vi "pneumatic control.vi"() -> ()   [LabVIEW 2018]
uses:
  <vilib>/Utility/error.llb/DialogType.ctl
  <vilib>/DAQmx/write.llb/DAQmx Write (Analog DBL 1Chan 1Samp).vi
  <vilib>/DAQmx/write.llb/DAQmx Write (Analog 1D DBL NChan 1Samp).vi
  <vilib>/DAQmx/create/channels.llb/DAQmx Create Channel (AO-Voltage-Basic).vi
  <vilib>/DAQmx/miscellaneous.llb/DAQmx Fill In Error Info.vi
panel:
  in  "水平指针滑动杆1-4":dbl(slide) scale=0.0..10.0
  in  "最大值 5":dbl=10.0 format="%0.2f"
  in  "无极控制停止按钮 1-4":bool
  in  "释放 1-4":bool
  in  "抓取1-4":bool
  in  "maximum value 6":dbl=10.0 caption="最大值" format="%0.2f"
  in  "抓放控制停止按钮1-4":bool
  in  "启用抓取控制1-4":bool
  in  "启用无极控制 1-4":bool
  in  "选项卡控件":enum32{"1-2-3", "1-3-4"}(tab)
  in  "水平指针滑动杆1-2-3":dbl(slide) scale=0.0..10.0
  in  "最大值 7":dbl=10.0 format="%0.2f"
  in  "无极控制停止按钮 1-2-3":bool
  in  "释放 1-2-3":bool
  in  "抓取1-2-3":bool
  in  "maximum value 8":dbl=10.0 caption="最大值" format="%0.2f"
  in  "抓放控制停止按钮1-2-3":bool
  in  "启用抓取控制1-2-3":bool
  in  "启用无极控制 1-2-3":bool
  in  "启用无极控制 1-3-4":bool
  in  "启用抓取控制1-3-4":bool
  in  "抓放控制停止按钮1-3-4":bool
  in  "maximum value 7":dbl=10.0 caption="最大值" format="%0.2f"
  in  "抓取1-3-4":bool
  in  "释放 1-3-4":bool
  in  "无极控制停止按钮 1-3-4":bool
  in  "最大值 6":dbl=10.0 format="%0.2f"
  in  "水平指针滑动杆1-3-4":dbl(slide) scale=0.0..10.0
  in  "水平指针滑动杆 4":dbl(slide) scale=0.0..10.0
  in  "最大值 4":dbl=10.0 format="%0.2f"
  in  "无极控制停止按钮 4":bool
  in  "释放 4":bool
  in  "抓取 4":bool
  in  "maximum value 5":dbl=10.0 caption="最大值" format="%0.2f"
  in  "抓放控制停止按钮 4":bool
  in  "启用抓取控制 4":bool
  in  "启用无极控制 4":bool
  in  "水平指针滑动杆 3":dbl(slide) scale=0.0..10.0
  in  "最大值 3":dbl=10.0 format="%0.2f"
  in  "无极控制停止按钮 3":bool
  in  "释放 3":bool
  in  "抓取 3":bool
  in  "maximum value 4":dbl=10.0 caption="最大值" format="%0.2f"
  in  "抓放控制停止按钮 3":bool
  in  "启用抓取控制 3":bool
  in  "启用无极控制 3":bool
  in  "水平指针滑动杆 2":dbl(slide) scale=0.0..10.0
  in  "最大值 2":dbl=10.0 format="%0.2f"
  in  "无极控制停止按钮 2":bool
  in  "释放 2":bool
  in  "抓取 2":bool
  in  "maximum value 3":dbl=10.0 caption="最大值" format="%0.2f"
  in  "抓放控制停止按钮 2":bool
  in  "启用抓取控制 2":bool
  in  "启用无极控制 2":bool
  in  "水平指针滑动杆":dbl(slide) scale=0.0..10.0
  in  "最大值":dbl=10.0 format="%0.2f"
  in  "无极控制停止按钮":bool
  in  "释放":bool
  in  "抓取":bool
  in  "maximum value 2":dbl=10.0 caption="最大值" format="%0.2f"
  in  "抓放控制停止按钮":bool
  in  "启用抓取控制":bool
  in  "启用无极控制":bool
  in  "总停止按钮":bool
  # "机械手驱动控制"
  # "机械手1抓放控制"
  # "机械手1滑条无极控制"
  # "机械手2抓放控制"
  # "机械手2滑条无极控制"
  # "机械手3抓放控制"
  # "机械手3滑条无极控制"
  # "机械手4抓放控制"
  # "机械手4滑条无极控制"
  # "机械手组合控制"
  # "机械手(1-4)一键控制"
  # "机械手抓放控制"
  # "机械手滑条无极控制"
  # "注意：\n  1、该模块共有“抓放控制”、“滑条无极控制”两种种机械手控制器。\n  2、点击任意控制器框内“启用X”按键即可启动该控制器，若需要切换控制器则需要先按下前面使用控制器“停止X”按键再按“启用X”按键。"
  # "机械手抓放控制"
  # "机械手滑条无极控制"
  # "机械手抓放控制"
  # "机械手滑条无极控制"
  # "4"
  # "3"
  # "2"
  # "1"
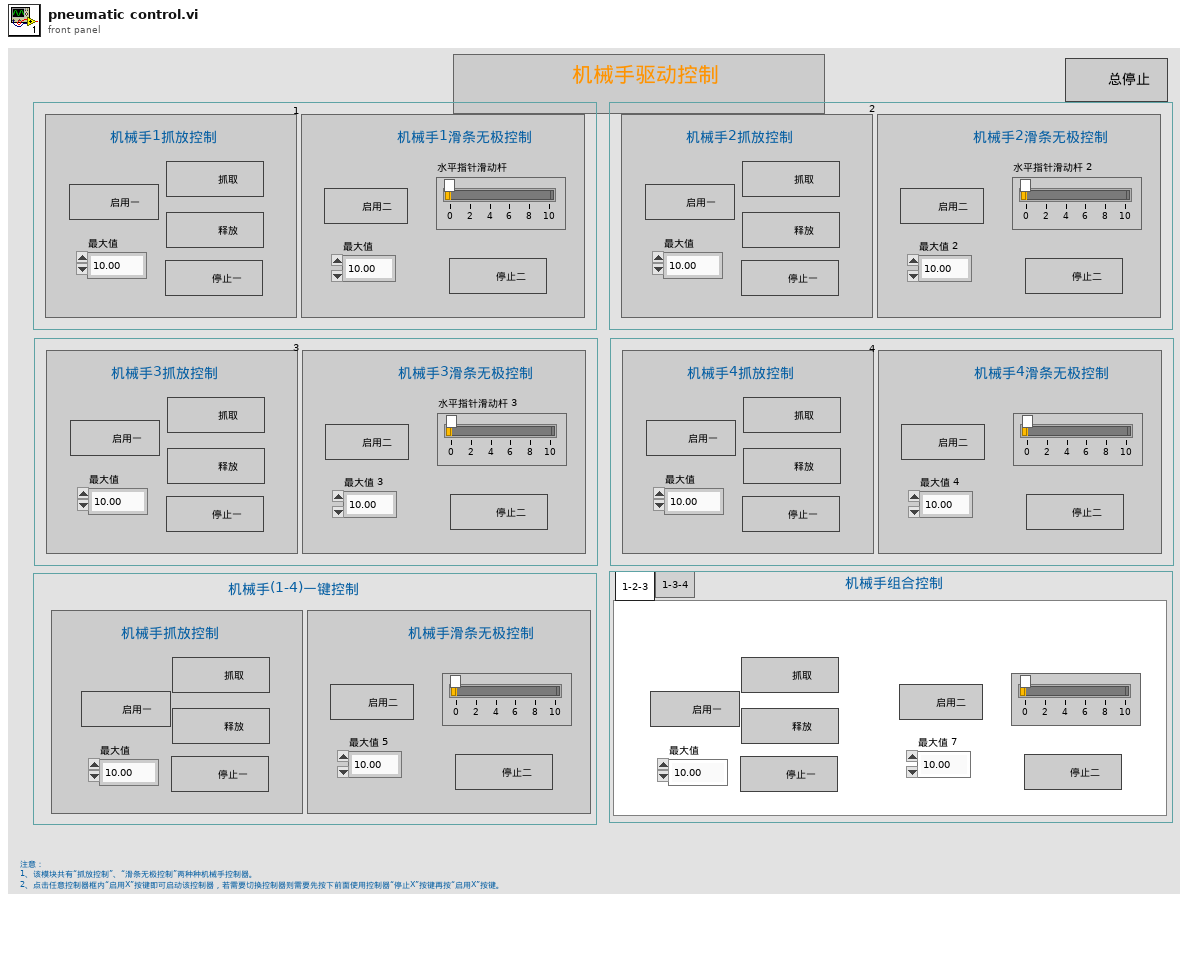
[diagram p1: front panel]
types:
  T1 = typedef "DialogType.ctl" = u16
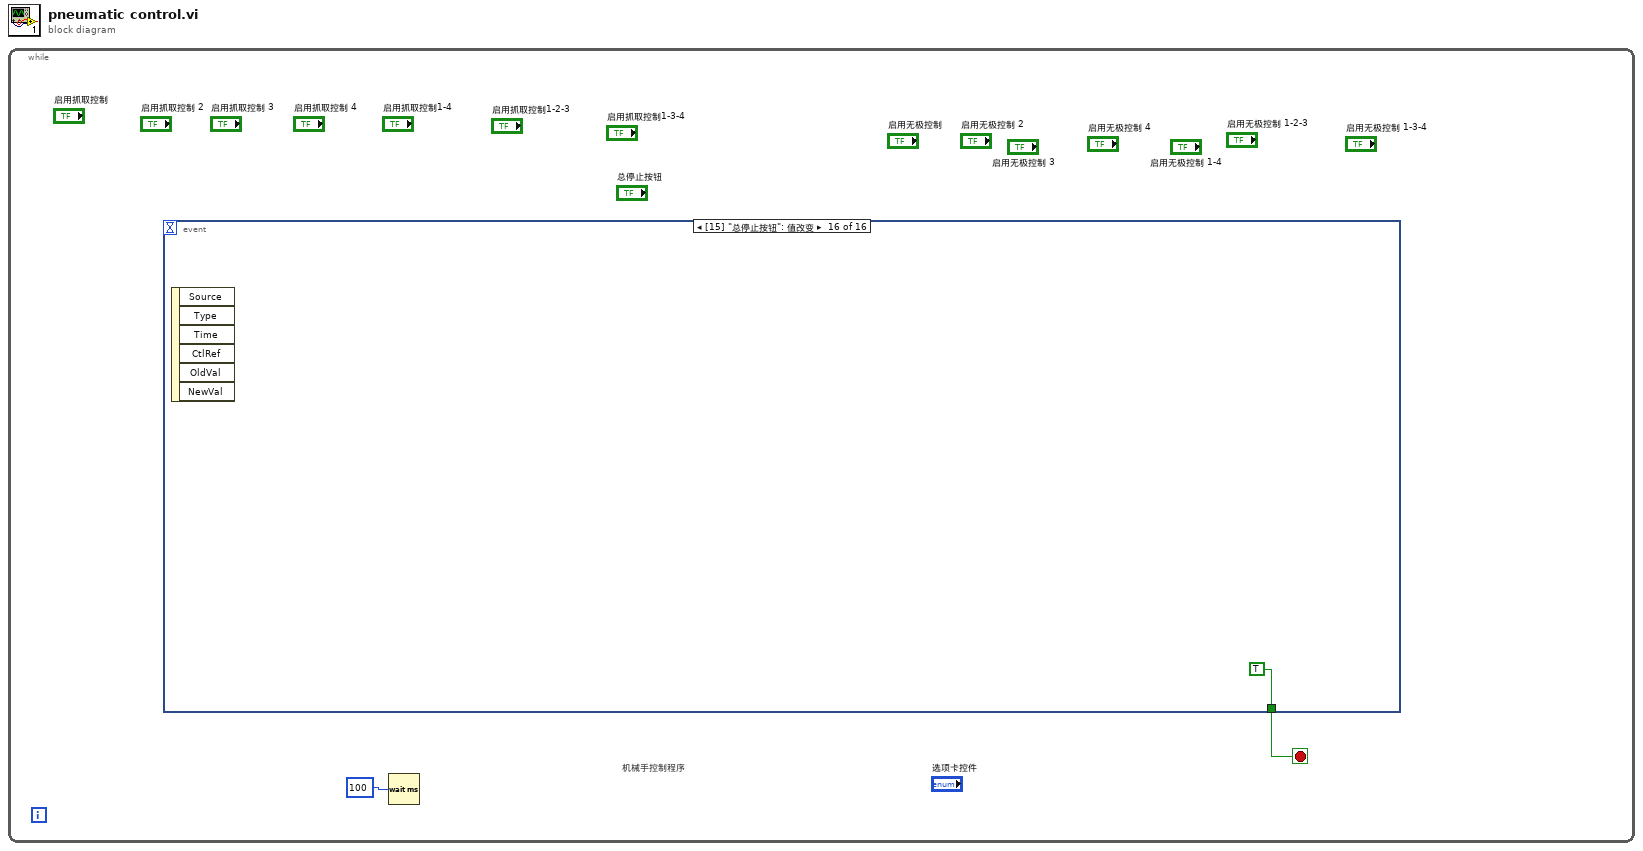
[diagram p0: block diagram]
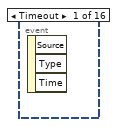
[diagram p2: hidden frame]
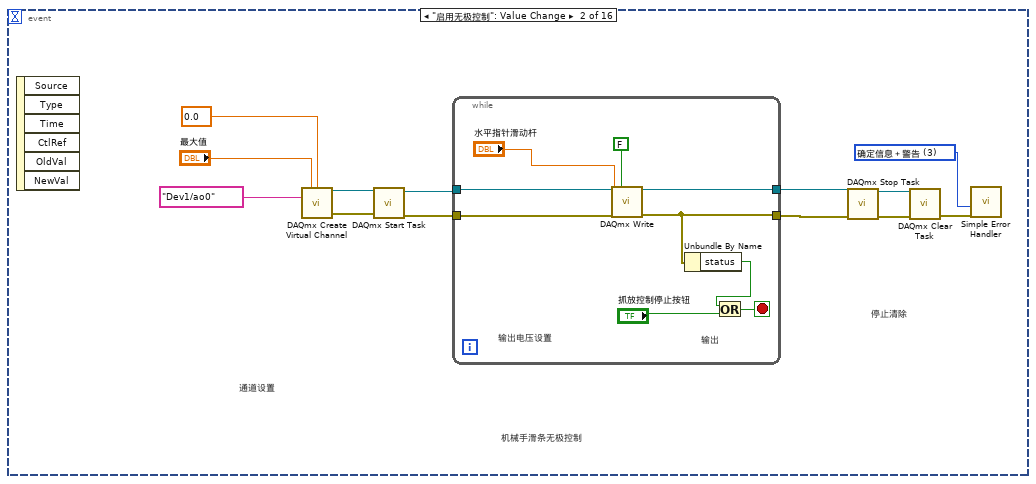
[diagram p3: hidden frame]
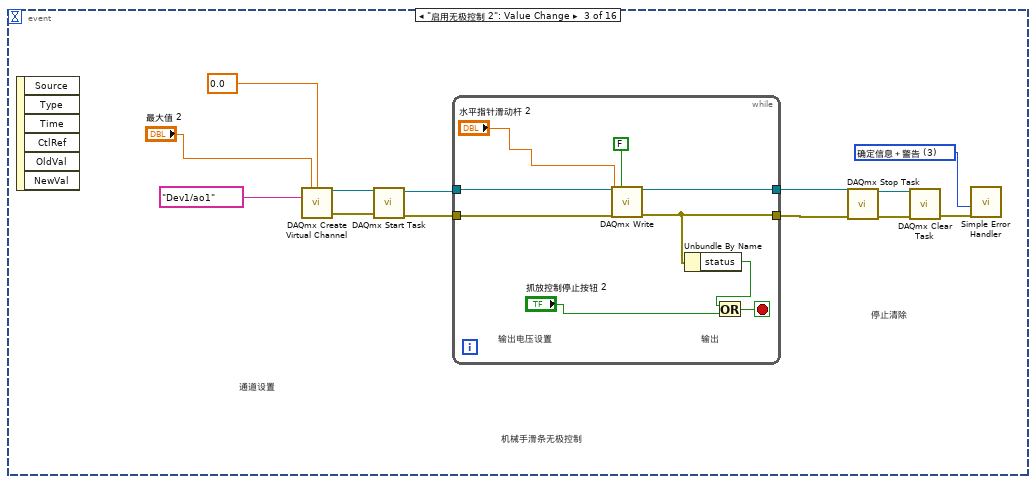
[diagram p4: hidden frame]
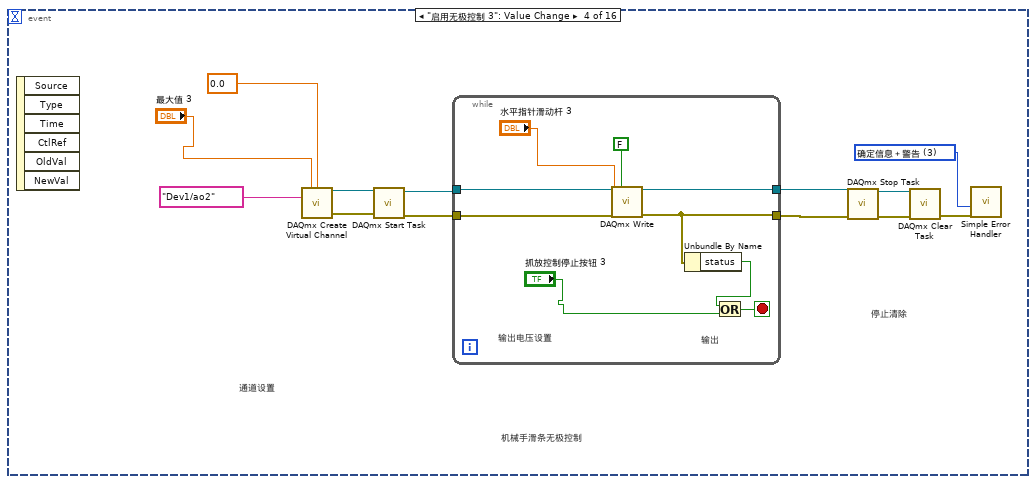
[diagram p5: hidden frame]
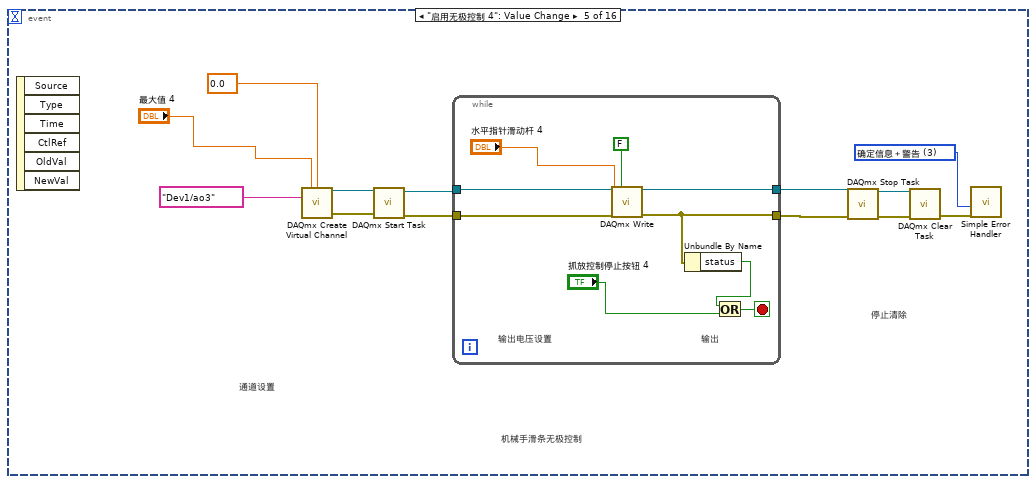
[diagram p6: hidden frame]
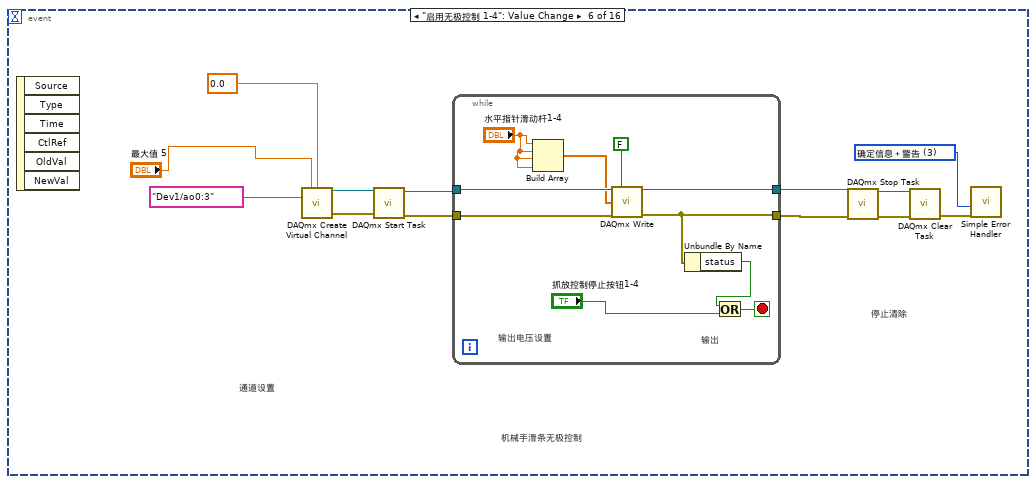
[diagram p7: hidden frame]
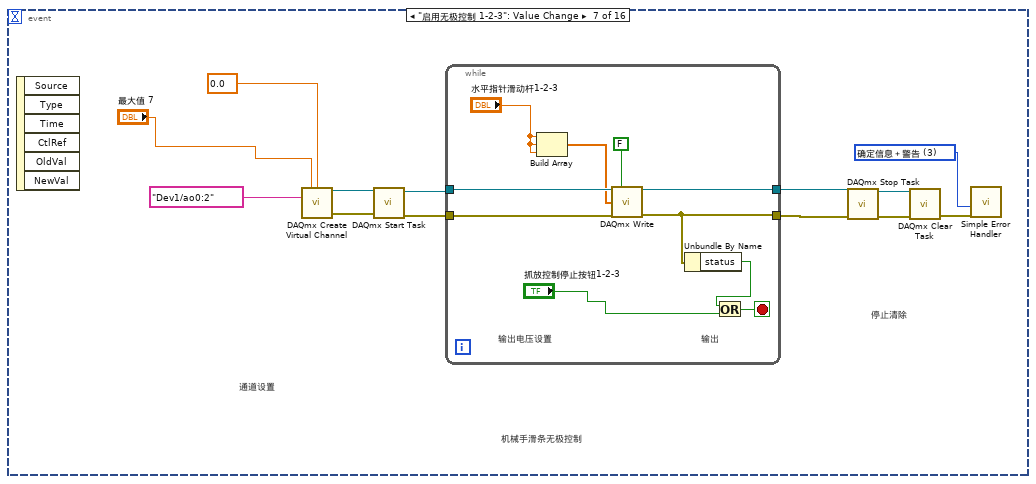
[diagram p8: hidden frame]
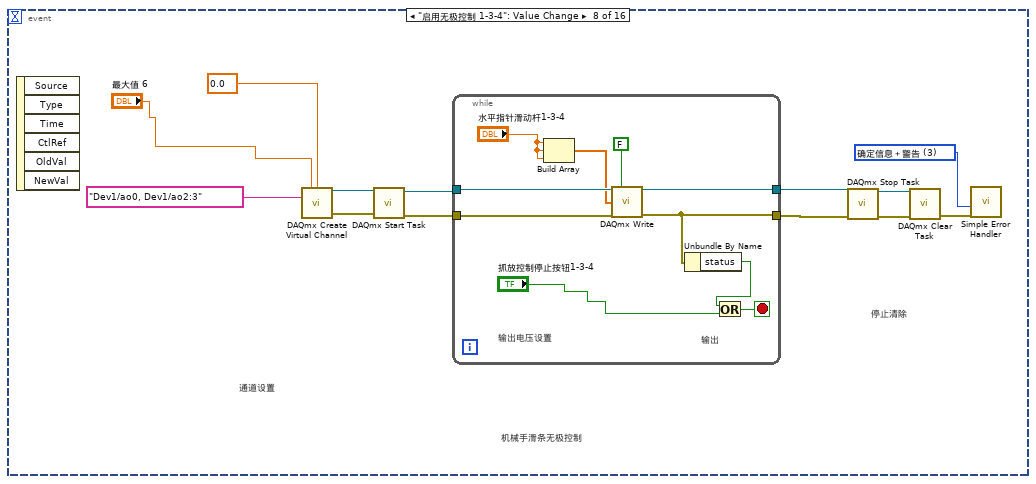
[diagram p9: hidden frame]
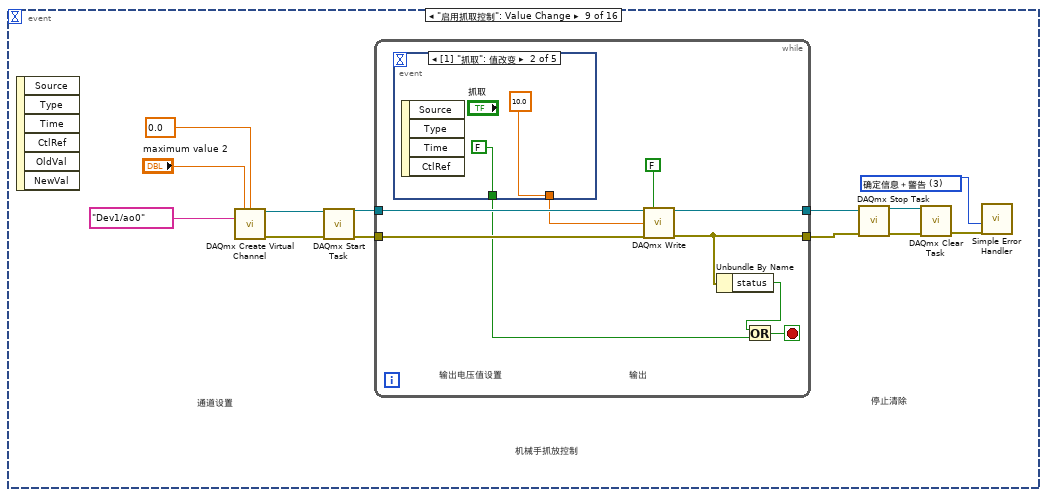
[diagram p10: hidden frame]
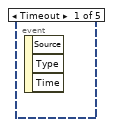
[diagram p11: hidden frame]
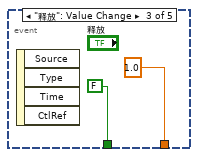
[diagram p12: hidden frame]
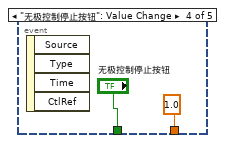
[diagram p13: hidden frame]
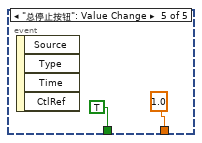
[diagram p14: hidden frame]
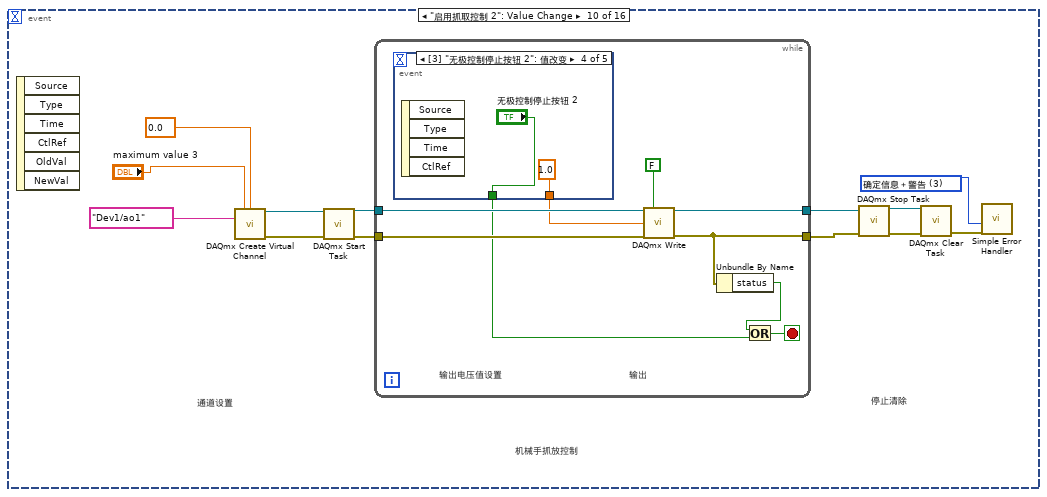
[diagram p15: hidden frame]
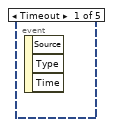
[diagram p16: hidden frame]
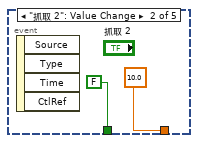
[diagram p17: hidden frame]
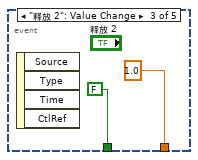
[diagram p18: hidden frame]
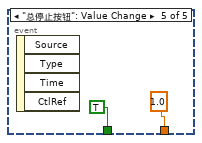
[diagram p19: hidden frame]
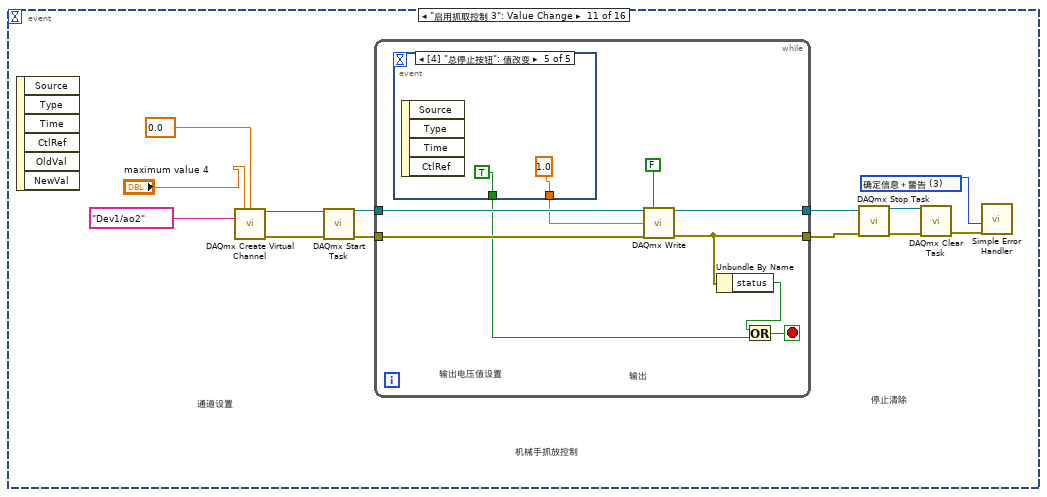
[diagram p20: hidden frame]
diagram:
  n1 = while {
    stop <- w1 stop-if-true
    # "机械手控制程序"
    n2 = event shown="[15] \"总停止按钮\": 值改变" {
      selector: _ -> [_ _ _ _ _ _ _ _ _ _ _ _ _ _ _ _]
      dyn-events: _ -> [_ _ _ _ _ _ _ _ _ _ _ _ _ _ _ _]
      timeout: _ -> [_ _ _ _ _ _ _ _ _ _ _ _ _ _ _ _]
      tunnel: [_ _ _ _ _ _ _ _ _ _ _ _ _ _ _ TRUE] -> w1
      event Timeout {
        n3 = event-data() -> ()  [unwired: 1 in, 3 out]
      }
      event "启用无极控制": Value Change {
        w4 = T1 3 items=["无对话框", "确定信息", "继续或停止信息", "确定信息＋警告", "继续/停止＋警告"] ("对话框类型（确定信息：1）")
        # "停止清除"
        # "通道设置"
        # "机械手滑条无极控制"
        n4 = event-data() -> ()  [unwired: 1 in, 6 out]
        n5 = call-poly <vilib>:"DAQmx Create Virtual Channel.vi"("maximum value"="最大值", "minimum value"=0.0, "physical channels"=tag "Dev1/ao0") -> ("task out"=w14:refnum<k21>, "error out"=w7:errorcluster)  [unwired: 11 in]
        n6 = call <vilib>:"DAQmx Start Task.vi"("task/channels in"=w14, "error in"=w7) -> ("task out"=w13:refnum<k21>, "error out"=w8:errorcluster)  [unwired: 12 in]
        n7 = while {
          tunnel: w13 -> [w24]
          tunnel: [w23] -> w12
          tunnel: w8 -> [w22]
          tunnel: [w20] -> w9
          stop <- w18 stop-if-true
          # "输出"
          # "输出电压设置"
          n8 = call-poly <vilib>:"DAQmx Write.vi"("task/channels in"=w24, "auto start"=FALSE, "data"="水平指针滑动杆", "error in"=w22) -> ("task out"=w23:refnum<k21>, "error out"=w20:errorcluster)  [unwired: 9 in, 1 out]
          n9 = Unbundle By Name(w20) -> ("status"=w19:bool)
          n10 = Or(x=w19, y="抓放控制停止按钮") -> (x .or. y?=w18:bool)
        }
        n11 = call <vilib>:"DAQmx Stop Task.vi"("task/channels in"=w12, "error in"=w9) -> ("task out"=w11:refnum<k21>, "error out"=w10:errorcluster)  [unwired: 12 in]
        n12 = call <vilib>:"DAQmx Clear Task.vi"("task in"=w11, "error in"=w10) -> ("error out"=w15:errorcluster)  [unwired: 13 in]
        n13 = call <vilib>:"Simple Error Handler.vi"("type of dialog (OK msg:1)"=w4, "error in (no error)"=w15) -> ()  [unwired: 3 in, 5 out]
      }
      event "启用无极控制 2": Value Change {
        w27 = T1 3 items=["无对话框", "确定信息", "继续或停止信息", "确定信息＋警告", "继续/停止＋警告"] ("对话框类型（确定信息：1）")
        # "停止清除"
        # "通道设置"
        # "机械手滑条无极控制"
        n14 = event-data() -> ()  [unwired: 1 in, 6 out]
        n15 = call-poly <vilib>:"DAQmx Create Virtual Channel.vi"("maximum value"="最大值 2", "minimum value"=0.0, "physical channels"=tag "Dev1/ao1") -> ("task out"=w36:refnum<k21>, "error out"=w29:errorcluster)  [unwired: 11 in]
        n16 = call <vilib>:"DAQmx Start Task.vi"("task/channels in"=w36, "error in"=w29) -> ("task out"=w35:refnum<k21>, "error out"=w30:errorcluster)  [unwired: 12 in]
        n17 = while {
          tunnel: w35 -> [w46]
          tunnel: [w45] -> w34
          tunnel: w30 -> [w44]
          tunnel: [w42] -> w31
          stop <- w40 stop-if-true
          # "输出"
          # "输出电压设置"
          n18 = call-poly <vilib>:"DAQmx Write.vi"("task/channels in"=w46, "auto start"=FALSE, "data"="水平指针滑动杆 2", "error in"=w44) -> ("task out"=w45:refnum<k21>, "error out"=w42:errorcluster)  [unwired: 9 in, 1 out]
          n19 = Unbundle By Name(w42) -> ("status"=w41:bool)
          n20 = Or(x=w41, y="抓放控制停止按钮 2") -> (x .or. y?=w40:bool)
        }
        n21 = call <vilib>:"DAQmx Stop Task.vi"("task/channels in"=w34, "error in"=w31) -> ("task out"=w33:refnum<k21>, "error out"=w32:errorcluster)  [unwired: 12 in]
        n22 = call <vilib>:"DAQmx Clear Task.vi"("task in"=w33, "error in"=w32) -> ("error out"=w37:errorcluster)  [unwired: 13 in]
        n23 = call <vilib>:"Simple Error Handler.vi"("type of dialog (OK msg:1)"=w27, "error in (no error)"=w37) -> ()  [unwired: 3 in, 5 out]
      }
      event "启用无极控制 3": Value Change {
        w49 = T1 3 items=["无对话框", "确定信息", "继续或停止信息", "确定信息＋警告", "继续/停止＋警告"] ("对话框类型（确定信息：1）")
        # "停止清除"
        # "通道设置"
        # "机械手滑条无极控制"
        n24 = event-data() -> ()  [unwired: 1 in, 6 out]
        n25 = call-poly <vilib>:"DAQmx Create Virtual Channel.vi"("maximum value"="最大值 3", "minimum value"=0.0, "physical channels"=tag "Dev1/ao2") -> ("task out"=w58:refnum<k21>, "error out"=w51:errorcluster)  [unwired: 11 in]
        n26 = call <vilib>:"DAQmx Start Task.vi"("task/channels in"=w58, "error in"=w51) -> ("task out"=w57:refnum<k21>, "error out"=w52:errorcluster)  [unwired: 12 in]
        n27 = while {
          tunnel: w57 -> [w68]
          tunnel: [w67] -> w56
          tunnel: w52 -> [w66]
          tunnel: [w64] -> w53
          stop <- w62 stop-if-true
          # "输出"
          # "输出电压设置"
          n28 = call-poly <vilib>:"DAQmx Write.vi"("task/channels in"=w68, "auto start"=FALSE, "data"="水平指针滑动杆 3", "error in"=w66) -> ("task out"=w67:refnum<k21>, "error out"=w64:errorcluster)  [unwired: 9 in, 1 out]
          n29 = Unbundle By Name(w64) -> ("status"=w63:bool)
          n30 = Or(x=w63, y="抓放控制停止按钮 3") -> (x .or. y?=w62:bool)
        }
        n31 = call <vilib>:"DAQmx Stop Task.vi"("task/channels in"=w56, "error in"=w53) -> ("task out"=w55:refnum<k21>, "error out"=w54:errorcluster)  [unwired: 12 in]
        n32 = call <vilib>:"DAQmx Clear Task.vi"("task in"=w55, "error in"=w54) -> ("error out"=w59:errorcluster)  [unwired: 13 in]
        n33 = call <vilib>:"Simple Error Handler.vi"("type of dialog (OK msg:1)"=w49, "error in (no error)"=w59) -> ()  [unwired: 3 in, 5 out]
      }
      event "启用无极控制 4": Value Change {
        w71 = T1 3 items=["无对话框", "确定信息", "继续或停止信息", "确定信息＋警告", "继续/停止＋警告"] ("对话框类型（确定信息：1）")
        # "停止清除"
        # "通道设置"
        # "机械手滑条无极控制"
        n34 = event-data() -> ()  [unwired: 1 in, 6 out]
        n35 = call-poly <vilib>:"DAQmx Create Virtual Channel.vi"("maximum value"="最大值 4", "minimum value"=0.0, "physical channels"=tag "Dev1/ao3") -> ("task out"=w80:refnum<k21>, "error out"=w73:errorcluster)  [unwired: 11 in]
        n36 = call <vilib>:"DAQmx Start Task.vi"("task/channels in"=w80, "error in"=w73) -> ("task out"=w79:refnum<k21>, "error out"=w74:errorcluster)  [unwired: 12 in]
        n37 = while {
          tunnel: w79 -> [w90]
          tunnel: [w89] -> w78
          tunnel: w74 -> [w88]
          tunnel: [w86] -> w75
          stop <- w84 stop-if-true
          # "输出"
          # "输出电压设置"
          n38 = call-poly <vilib>:"DAQmx Write.vi"("task/channels in"=w90, "auto start"=FALSE, "data"="水平指针滑动杆 4", "error in"=w88) -> ("task out"=w89:refnum<k21>, "error out"=w86:errorcluster)  [unwired: 9 in, 1 out]
          n39 = Unbundle By Name(w86) -> ("status"=w85:bool)
          n40 = Or(x=w85, y="抓放控制停止按钮 4") -> (x .or. y?=w84:bool)
        }
        n41 = call <vilib>:"DAQmx Stop Task.vi"("task/channels in"=w78, "error in"=w75) -> ("task out"=w77:refnum<k21>, "error out"=w76:errorcluster)  [unwired: 12 in]
        n42 = call <vilib>:"DAQmx Clear Task.vi"("task in"=w77, "error in"=w76) -> ("error out"=w81:errorcluster)  [unwired: 13 in]
        n43 = call <vilib>:"Simple Error Handler.vi"("type of dialog (OK msg:1)"=w71, "error in (no error)"=w81) -> ()  [unwired: 3 in, 5 out]
      }
      event "启用无极控制 1-4": Value Change {
        w93 = T1 3 items=["无对话框", "确定信息", "继续或停止信息", "确定信息＋警告", "继续/停止＋警告"] ("对话框类型（确定信息：1）")
        # "停止清除"
        # "通道设置"
        # "机械手滑条无极控制"
        n44 = event-data() -> ()  [unwired: 1 in, 6 out]
        n45 = call-poly <vilib>:"DAQmx Create Virtual Channel.vi"("maximum value"="最大值 5", "minimum value"=0.0, "physical channels"=tag "Dev1/ao0:3") -> ("task out"=w102:refnum<k21>, "error out"=w95:errorcluster)  [unwired: 11 in]
        n46 = call <vilib>:"DAQmx Start Task.vi"("task/channels in"=w102, "error in"=w95) -> ("task out"=w101:refnum<k21>, "error out"=w96:errorcluster)  [unwired: 12 in]
        n47 = while {
          tunnel: w101 -> [w113]
          tunnel: [w112] -> w100
          tunnel: w96 -> [w111]
          tunnel: [w109] -> w97
          stop <- w107 stop-if-true
          # "输出"
          # "输出电压设置"
          n48 = Build Array("水平指针滑动杆1-4", "水平指针滑动杆1-4", "水平指针滑动杆1-4", "水平指针滑动杆1-4") -> (w104:dbl[])
          n49 = call-poly <vilib>:"DAQmx Write.vi"("task/channels in"=w113, "auto start"=FALSE, "data"=w104, "error in"=w111) -> ("task out"=w112:refnum<k21>, "error out"=w109:errorcluster)  [unwired: 9 in, 1 out]
          n50 = Unbundle By Name(w109) -> ("status"=w108:bool)
          n51 = Or(x=w108, y="抓放控制停止按钮1-4") -> (x .or. y?=w107:bool)
        }
        n52 = call <vilib>:"DAQmx Stop Task.vi"("task/channels in"=w100, "error in"=w97) -> ("task out"=w99:refnum<k21>, "error out"=w98:errorcluster)  [unwired: 12 in]
        n53 = call <vilib>:"DAQmx Clear Task.vi"("task in"=w99, "error in"=w98) -> ("error out"=w103:errorcluster)  [unwired: 13 in]
        n54 = call <vilib>:"Simple Error Handler.vi"("type of dialog (OK msg:1)"=w93, "error in (no error)"=w103) -> ()  [unwired: 3 in, 5 out]
      }
      event "启用无极控制 1-2-3": Value Change {
        w116 = T1 3 items=["无对话框", "确定信息", "继续或停止信息", "确定信息＋警告", "继续/停止＋警告"] ("对话框类型（确定信息：1）")
        # "停止清除"
        # "通道设置"
        # "机械手滑条无极控制"
        n55 = event-data() -> ()  [unwired: 1 in, 6 out]
        n56 = call-poly <vilib>:"DAQmx Create Virtual Channel.vi"("maximum value"="最大值 7", "minimum value"=0.0, "physical channels"=tag "Dev1/ao0:2") -> ("task out"=w125:refnum<k21>, "error out"=w118:errorcluster)  [unwired: 11 in]
        n57 = call <vilib>:"DAQmx Start Task.vi"("task/channels in"=w125, "error in"=w118) -> ("task out"=w124:refnum<k21>, "error out"=w119:errorcluster)  [unwired: 12 in]
        n58 = while {
          tunnel: w124 -> [w136]
          tunnel: [w135] -> w123
          tunnel: w119 -> [w134]
          tunnel: [w132] -> w120
          stop <- w130 stop-if-true
          # "输出"
          # "输出电压设置"
          n59 = Build Array("水平指针滑动杆1-2-3", "水平指针滑动杆1-2-3", "水平指针滑动杆1-2-3") -> (w127:dbl[])
          n60 = call-poly <vilib>:"DAQmx Write.vi"("task/channels in"=w136, "auto start"=FALSE, "data"=w127, "error in"=w134) -> ("task out"=w135:refnum<k21>, "error out"=w132:errorcluster)  [unwired: 9 in, 1 out]
          n61 = Unbundle By Name(w132) -> ("status"=w131:bool)
          n62 = Or(x=w131, y="抓放控制停止按钮1-2-3") -> (x .or. y?=w130:bool)
        }
        n63 = call <vilib>:"DAQmx Stop Task.vi"("task/channels in"=w123, "error in"=w120) -> ("task out"=w122:refnum<k21>, "error out"=w121:errorcluster)  [unwired: 12 in]
        n64 = call <vilib>:"DAQmx Clear Task.vi"("task in"=w122, "error in"=w121) -> ("error out"=w126:errorcluster)  [unwired: 13 in]
        n65 = call <vilib>:"Simple Error Handler.vi"("type of dialog (OK msg:1)"=w116, "error in (no error)"=w126) -> ()  [unwired: 3 in, 5 out]
      }
      event "启用无极控制 1-3-4": Value Change {
        w139 = T1 3 items=["无对话框", "确定信息", "继续或停止信息", "确定信息＋警告", "继续/停止＋警告"] ("对话框类型（确定信息：1）")
        # "停止清除"
        # "通道设置"
        # "机械手滑条无极控制"
        n66 = event-data() -> ()  [unwired: 1 in, 6 out]
        n67 = call-poly <vilib>:"DAQmx Create Virtual Channel.vi"("maximum value"="最大值 6", "minimum value"=0.0, "physical channels"=tag "Dev1/ao0, Dev1/ao2:3") -> ("task out"=w148:refnum<k21>, "error out"=w141:errorcluster)  [unwired: 11 in]
        n68 = call <vilib>:"DAQmx Start Task.vi"("task/channels in"=w148, "error in"=w141) -> ("task out"=w147:refnum<k21>, "error out"=w142:errorcluster)  [unwired: 12 in]
        n69 = while {
          tunnel: w147 -> [w159]
          tunnel: [w158] -> w146
          tunnel: w142 -> [w157]
          tunnel: [w155] -> w143
          stop <- w153 stop-if-true
          # "输出"
          # "输出电压设置"
          n70 = Build Array("水平指针滑动杆1-3-4", "水平指针滑动杆1-3-4", "水平指针滑动杆1-3-4") -> (w150:dbl[])
          n71 = call-poly <vilib>:"DAQmx Write.vi"("task/channels in"=w159, "auto start"=FALSE, "data"=w150, "error in"=w157) -> ("task out"=w158:refnum<k21>, "error out"=w155:errorcluster)  [unwired: 9 in, 1 out]
          n72 = Unbundle By Name(w155) -> ("status"=w154:bool)
          n73 = Or(x=w154, y="抓放控制停止按钮1-3-4") -> (x .or. y?=w153:bool)
        }
        n74 = call <vilib>:"DAQmx Stop Task.vi"("task/channels in"=w146, "error in"=w143) -> ("task out"=w145:refnum<k21>, "error out"=w144:errorcluster)  [unwired: 12 in]
        n75 = call <vilib>:"DAQmx Clear Task.vi"("task in"=w145, "error in"=w144) -> ("error out"=w149:errorcluster)  [unwired: 13 in]
        n76 = call <vilib>:"Simple Error Handler.vi"("type of dialog (OK msg:1)"=w139, "error in (no error)"=w149) -> ()  [unwired: 3 in, 5 out]
      }
      event "启用抓取控制": Value Change {
        w161 = T1 3 items=["无对话框", "确定信息", "继续或停止信息", "确定信息＋警告", "继续/停止＋警告"] ("对话框类型（确定信息：1）")
        # "停止清除"
        # "通道设置"
        # "机械手抓放控制"
        n77 = event-data() -> ()  [unwired: 1 in, 6 out]
        n78 = call-poly <vilib>:"DAQmx Create Virtual Channel.vi"("maximum value"="maximum value 2", "minimum value"=0.0 ("minimum value 2"), "physical channels"=tag "Dev1/ao0") -> ("task out"=w163:refnum<k21>, "error out"=w170:errorcluster)  [unwired: 11 in]
        n79 = call <vilib>:"DAQmx Start Task.vi"("task/channels in"=w163, "error in"=w170) -> ("task out"=w164:refnum<k21>, "error out"=w169:errorcluster)  [unwired: 12 in]
        n80 = while {
          tunnel: w164 -> [w181]
          tunnel: [w180] -> w165
          tunnel: w169 -> [w179]
          tunnel: [w177] -> w168
          stop <- w175 stop-if-true
          # "输出"
          # "输出电压值设置"
          n81 = event shown="[1] \"抓取\": 值改变" {
            selector: _ -> [_ _ _ _ _]
            dyn-events: _ -> [_ _ _ _ _]
            timeout: _ -> [_ _ _ _ _]
            tunnel: [_ 10.0 ("data") 1.0 ("data") 1.0 ("data") 1.0 ("data")] -> w174
            tunnel: [_ FALSE FALSE "无极控制停止按钮" TRUE] -> w173
            event Timeout {
              n82 = event-data() -> ()  [unwired: 1 in, 3 out]
            }
            event "抓取": Value Change {
              n83 = event-data() -> ()  [unwired: 1 in, 4 out]
            }
            event "释放": Value Change {
              n84 = event-data() -> ()  [unwired: 1 in, 4 out]
            }
            event "无极控制停止按钮": Value Change {
              n85 = event-data() -> ()  [unwired: 1 in, 4 out]
            }
            event "总停止按钮": Value Change {
              n86 = event-data() -> ()  [unwired: 1 in, 4 out]
            }
          }
          n87 = call-poly <vilib>:"DAQmx Write.vi"("task/channels in"=w181, "auto start"=FALSE, "data"=w174, "error in"=w179) -> ("task out"=w180:refnum<k21>, "error out"=w177:errorcluster)  [unwired: 9 in, 1 out]
          n88 = Unbundle By Name(w177) -> ("status"=w176:bool)
          n89 = Or(x=w176, y=w173) -> (x .or. y?=w175:bool)
        }
        n90 = call <vilib>:"DAQmx Stop Task.vi"("task/channels in"=w165, "error in"=w168) -> ("task out"=w166:refnum<k21>, "error out"=w167:errorcluster)  [unwired: 12 in]
        n91 = call <vilib>:"DAQmx Clear Task.vi"("task in"=w166, "error in"=w167) -> ("error out"=w162:errorcluster)  [unwired: 13 in]
        n92 = call <vilib>:"Simple Error Handler.vi"("type of dialog (OK msg:1)"=w161, "error in (no error)"=w162) -> ()  [unwired: 3 in, 5 out]
      }
      event "启用抓取控制 2": Value Change {
        w192 = T1 3 items=["无对话框", "确定信息", "继续或停止信息", "确定信息＋警告", "继续/停止＋警告"] ("对话框类型（确定信息：1）")
        # "停止清除"
        # "通道设置"
        # "机械手抓放控制"
        n93 = event-data() -> ()  [unwired: 1 in, 6 out]
        n94 = call-poly <vilib>:"DAQmx Create Virtual Channel.vi"("maximum value"="maximum value 3", "minimum value"=0.0 ("minimum value 2"), "physical channels"=tag "Dev1/ao1") -> ("task out"=w194:refnum<k21>, "error out"=w201:errorcluster)  [unwired: 11 in]
        n95 = call <vilib>:"DAQmx Start Task.vi"("task/channels in"=w194, "error in"=w201) -> ("task out"=w195:refnum<k21>, "error out"=w200:errorcluster)  [unwired: 12 in]
        n96 = while {
          tunnel: w195 -> [w211]
          tunnel: [w210] -> w196
          tunnel: w200 -> [w209]
          tunnel: [w207] -> w199
          stop <- w205 stop-if-true
          # "输出"
          # "输出电压值设置"
          n97 = event shown="[3] \"无极控制停止按钮 2\": 值改变" {
            selector: _ -> [_ _ _ _ _]
            dyn-events: _ -> [_ _ _ _ _]
            timeout: _ -> [_ _ _ _ _]
            tunnel: [_ 10.0 ("data") 1.0 ("data") 1.0 ("data") 1.0 ("data")] -> w204
            tunnel: [_ FALSE FALSE "无极控制停止按钮 2" TRUE] -> w203
            event Timeout {
              n98 = event-data() -> ()  [unwired: 1 in, 3 out]
            }
            event "抓取 2": Value Change {
              n99 = event-data() -> ()  [unwired: 1 in, 4 out]
            }
            event "释放 2": Value Change {
              n100 = event-data() -> ()  [unwired: 1 in, 4 out]
            }
            event "无极控制停止按钮 2": Value Change {
              n101 = event-data() -> ()  [unwired: 1 in, 4 out]
            }
            event "总停止按钮": Value Change {
              n102 = event-data() -> ()  [unwired: 1 in, 4 out]
            }
          }
          n103 = call-poly <vilib>:"DAQmx Write.vi"("task/channels in"=w211, "auto start"=FALSE, "data"=w204, "error in"=w209) -> ("task out"=w210:refnum<k21>, "error out"=w207:errorcluster)  [unwired: 9 in, 1 out]
          n104 = Unbundle By Name(w207) -> ("status"=w206:bool)
          n105 = Or(x=w206, y=w203) -> (x .or. y?=w205:bool)
        }
        n106 = call <vilib>:"DAQmx Stop Task.vi"("task/channels in"=w196, "error in"=w199) -> ("task out"=w197:refnum<k21>, "error out"=w198:errorcluster)  [unwired: 12 in]
        n107 = call <vilib>:"DAQmx Clear Task.vi"("task in"=w197, "error in"=w198) -> ("error out"=w193:errorcluster)  [unwired: 13 in]
        n108 = call <vilib>:"Simple Error Handler.vi"("type of dialog (OK msg:1)"=w192, "error in (no error)"=w193) -> ()  [unwired: 3 in, 5 out]
      }
      event "启用抓取控制 3": Value Change {
        w222 = T1 3 items=["无对话框", "确定信息", "继续或停止信息", "确定信息＋警告", "继续/停止＋警告"] ("对话框类型（确定信息：1）")
        # "停止清除"
        # "通道设置"
        # "机械手抓放控制"
        n109 = event-data() -> ()  [unwired: 1 in, 6 out]
        n110 = call-poly <vilib>:"DAQmx Create Virtual Channel.vi"("maximum value"="maximum value 4", "minimum value"=0.0 ("minimum value 2"), "physical channels"=tag "Dev1/ao2") -> ("task out"=w224:refnum<k21>, "error out"=w231:errorcluster)  [unwired: 11 in]
        n111 = call <vilib>:"DAQmx Start Task.vi"("task/channels in"=w224, "error in"=w231) -> ("task out"=w225:refnum<k21>, "error out"=w230:errorcluster)  [unwired: 12 in]
        n112 = while {
          tunnel: w225 -> [w241]
          tunnel: [w240] -> w226
          tunnel: w230 -> [w239]
          tunnel: [w237] -> w229
          stop <- w235 stop-if-true
          # "输出"
          # "输出电压值设置"
          n113 = event shown="[4] \"总停止按钮\": 值改变" {
            selector: _ -> [_ _ _ _ _]
            dyn-events: _ -> [_ _ _ _ _]
            timeout: _ -> [_ _ _ _ _]
            tunnel: [_ 10.0 ("data") 1.0 ("data") 1.0 ("data") 1.0 ("data")] -> w234
            tunnel: [_ FALSE FALSE "无极控制停止按钮 3" TRUE] -> w233
            event Timeout {
              n114 = event-data() -> ()  [unwired: 1 in, 3 out]
            }
            event "抓取 3": Value Change {
              n115 = event-data() -> ()  [unwired: 1 in, 4 out]
            }
            event "释放 3": Value Change {
              n116 = event-data() -> ()  [unwired: 1 in, 4 out]
            }
            event "无极控制停止按钮 3": Value Change {
              n117 = event-data() -> ()  [unwired: 1 in, 4 out]
            }
            event "总停止按钮": Value Change {
              n118 = event-data() -> ()  [unwired: 1 in, 4 out]
            }
          }
          n119 = call-poly <vilib>:"DAQmx Write.vi"("task/channels in"=w241, "auto start"=FALSE, "data"=w234, "error in"=w239) -> ("task out"=w240:refnum<k21>, "error out"=w237:errorcluster)  [unwired: 9 in, 1 out]
          n120 = Unbundle By Name(w237) -> ("status"=w236:bool)
          n121 = Or(x=w236, y=w233) -> (x .or. y?=w235:bool)
        }
        n122 = call <vilib>:"DAQmx Stop Task.vi"("task/channels in"=w226, "error in"=w229) -> ("task out"=w227:refnum<k21>, "error out"=w228:errorcluster)  [unwired: 12 in]
        n123 = call <vilib>:"DAQmx Clear Task.vi"("task in"=w227, "error in"=w228) -> ("error out"=w223:errorcluster)  [unwired: 13 in]
        n124 = call <vilib>:"Simple Error Handler.vi"("type of dialog (OK msg:1)"=w222, "error in (no error)"=w223) -> ()  [unwired: 3 in, 5 out]
      }
      event "启用抓取控制 4": Value Change {
        w252 = T1 3 items=["无对话框", "确定信息", "继续或停止信息", "确定信息＋警告", "继续/停止＋警告"] ("对话框类型（确定信息：1）")
        # "停止清除"
        # "通道设置"
        # "机械手抓放控制"
        n125 = event-data() -> ()  [unwired: 1 in, 6 out]
        n126 = call-poly <vilib>:"DAQmx Create Virtual Channel.vi"("maximum value"="maximum value 5", "minimum value"=0.0 ("minimum value 2"), "physical channels"=tag "Dev1/ao3") -> ("task out"=w254:refnum<k21>, "error out"=w261:errorcluster)  [unwired: 11 in]
        n127 = call <vilib>:"DAQmx Start Task.vi"("task/channels in"=w254, "error in"=w261) -> ("task out"=w255:refnum<k21>, "error out"=w260:errorcluster)  [unwired: 12 in]
        n128 = while {
          tunnel: w255 -> [w271]
          tunnel: [w270] -> w256
          tunnel: w260 -> [w269]
          tunnel: [w267] -> w259
          stop <- w265 stop-if-true
          # "输出"
          # "输出电压值设置"
          n129 = event shown="[3] \"无极控制停止按钮 4\": 值改变" {
            selector: _ -> [_ _ _ _ _]
            dyn-events: _ -> [_ _ _ _ _]
            timeout: _ -> [_ _ _ _ _]
            tunnel: [_ 10.0 ("data") 1.0 ("data") 1.0 ("data") 1.0 ("data")] -> w264
            tunnel: [_ FALSE FALSE "无极控制停止按钮 4" TRUE] -> w263
            event Timeout {
              n130 = event-data() -> ()  [unwired: 1 in, 3 out]
            }
            event "抓取 4": Value Change {
              n131 = event-data() -> ()  [unwired: 1 in, 4 out]
            }
            event "释放 4": Value Change {
              n132 = event-data() -> ()  [unwired: 1 in, 4 out]
            }
            event "无极控制停止按钮 4": Value Change {
              n133 = event-data() -> ()  [unwired: 1 in, 4 out]
            }
            event "总停止按钮": Value Change {
              n134 = event-data() -> ()  [unwired: 1 in, 4 out]
            }
          }
          n135 = call-poly <vilib>:"DAQmx Write.vi"("task/channels in"=w271, "auto start"=FALSE, "data"=w264, "error in"=w269) -> ("task out"=w270:refnum<k21>, "error out"=w267:errorcluster)  [unwired: 9 in, 1 out]
          n136 = Unbundle By Name(w267) -> ("status"=w266:bool)
          n137 = Or(x=w266, y=w263) -> (x .or. y?=w265:bool)
        }
        n138 = call <vilib>:"DAQmx Stop Task.vi"("task/channels in"=w256, "error in"=w259) -> ("task out"=w257:refnum<k21>, "error out"=w258:errorcluster)  [unwired: 12 in]
        n139 = call <vilib>:"DAQmx Clear Task.vi"("task in"=w257, "error in"=w258) -> ("error out"=w253:errorcluster)  [unwired: 13 in]
        n140 = call <vilib>:"Simple Error Handler.vi"("type of dialog (OK msg:1)"=w252, "error in (no error)"=w253) -> ()  [unwired: 3 in, 5 out]
      }
      event "启用抓取控制1-4": Value Change {
        w282 = T1 3 items=["无对话框", "确定信息", "继续或停止信息", "确定信息＋警告", "继续/停止＋警告"] ("对话框类型（确定信息：1）")
        # "停止清除"
        # "通道设置"
        # "机械手抓放控制"
        n141 = event-data() -> ()  [unwired: 1 in, 6 out]
        n142 = call-poly <vilib>:"DAQmx Create Virtual Channel.vi"("maximum value"="maximum value 6", "minimum value"=0.0 ("minimum value 2"), "physical channels"=tag "Dev1/ao0:3") -> ("task out"=w284:refnum<k21>, "error out"=w291:errorcluster)  [unwired: 11 in]
        n143 = call <vilib>:"DAQmx Start Task.vi"("task/channels in"=w284, "error in"=w291) -> ("task out"=w285:refnum<k21>, "error out"=w290:errorcluster)  [unwired: 12 in]
        n144 = while {
          tunnel: w285 -> [w302]
          tunnel: [w301] -> w286
          tunnel: w290 -> [w300]
          tunnel: [w298] -> w289
          stop <- w296 stop-if-true
          # "输出"
          # "输出电压值设置"
          n145 = event shown="[3] \"无极控制停止按钮 1-4\": 值改变" {
            selector: _ -> [_ _ _ _ _]
            dyn-events: _ -> [_ _ _ _ _]
            timeout: _ -> [_ _ _ _ _]
            tunnel: [_ 10.0 ("data") 1.0 ("data") 1.0 ("data") 1.0 ("data")] -> w294
            tunnel: [_ FALSE FALSE "无极控制停止按钮 1-4" TRUE] -> w295
            event Timeout {
              n146 = event-data() -> ()  [unwired: 1 in, 3 out]
            }
            event "抓取1-4": Value Change {
              n147 = event-data() -> ()  [unwired: 1 in, 4 out]
            }
            event "释放 1-4": Value Change {
              n148 = event-data() -> ()  [unwired: 1 in, 4 out]
            }
            event "无极控制停止按钮 1-4": Value Change {
              n149 = event-data() -> ()  [unwired: 1 in, 4 out]
            }
            event "总停止按钮": Value Change {
              n150 = event-data() -> ()  [unwired: 1 in, 4 out]
            }
          }
          n151 = Build Array(w294, w294, w294, w294) -> (w293:dbl[])
          n152 = call-poly <vilib>:"DAQmx Write.vi"("task/channels in"=w302, "auto start"=FALSE, "data"=w293, "error in"=w300) -> ("task out"=w301:refnum<k21>, "error out"=w298:errorcluster)  [unwired: 9 in, 1 out]
          n153 = Unbundle By Name(w298) -> ("status"=w297:bool)
          n154 = Or(x=w297, y=w295) -> (x .or. y?=w296:bool)
        }
        n155 = call <vilib>:"DAQmx Stop Task.vi"("task/channels in"=w286, "error in"=w289) -> ("task out"=w287:refnum<k21>, "error out"=w288:errorcluster)  [unwired: 12 in]
        n156 = call <vilib>:"DAQmx Clear Task.vi"("task in"=w287, "error in"=w288) -> ("error out"=w283:errorcluster)  [unwired: 13 in]
        n157 = call <vilib>:"Simple Error Handler.vi"("type of dialog (OK msg:1)"=w282, "error in (no error)"=w283) -> ()  [unwired: 3 in, 5 out]
      }
      event "启用抓取控制1-2-3": Value Change {
        w313 = T1 3 items=["无对话框", "确定信息", "继续或停止信息", "确定信息＋警告", "继续/停止＋警告"] ("对话框类型（确定信息：1）")
        # "停止清除"
        # "通道设置"
        # "机械手抓放控制"
        n158 = event-data() -> ()  [unwired: 1 in, 6 out]
        n159 = call-poly <vilib>:"DAQmx Create Virtual Channel.vi"("maximum value"="maximum value 8", "minimum value"=0.0 ("minimum value 2"), "physical channels"=tag "Dev1/ao0:2") -> ("task out"=w315:refnum<k21>, "error out"=w322:errorcluster)  [unwired: 11 in]
        n160 = call <vilib>:"DAQmx Start Task.vi"("task/channels in"=w315, "error in"=w322) -> ("task out"=w316:refnum<k21>, "error out"=w321:errorcluster)  [unwired: 12 in]
        n161 = while {
          tunnel: w316 -> [w333]
          tunnel: [w332] -> w317
          tunnel: w321 -> [w331]
          tunnel: [w329] -> w320
          stop <- w327 stop-if-true
          # "输出"
          # "输出电压值设置"
          n162 = event shown="[3] \"无极控制停止按钮 1-2-3\": 值改变" {
            selector: _ -> [_ _ _ _ _]
            dyn-events: _ -> [_ _ _ _ _]
            timeout: _ -> [_ _ _ _ _]
            tunnel: [_ 10.0 ("data") 1.0 ("data") 1.0 ("data") 1.0 ("data")] -> w325
            tunnel: [_ FALSE FALSE "无极控制停止按钮 1-2-3" TRUE] -> w326
            event Timeout {
              n163 = event-data() -> ()  [unwired: 1 in, 3 out]
            }
            event "抓取1-2-3": Value Change {
              n164 = event-data() -> ()  [unwired: 1 in, 4 out]
            }
            event "释放 1-2-3": Value Change {
              n165 = event-data() -> ()  [unwired: 1 in, 4 out]
            }
            event "无极控制停止按钮 1-2-3": Value Change {
              n166 = event-data() -> ()  [unwired: 1 in, 4 out]
            }
            event "总停止按钮": Value Change {
              n167 = event-data() -> ()  [unwired: 1 in, 4 out]
            }
          }
          n168 = Build Array(w325, w325, w325) -> (w324:dbl[])
          n169 = call-poly <vilib>:"DAQmx Write.vi"("task/channels in"=w333, "auto start"=FALSE, "data"=w324, "error in"=w331) -> ("task out"=w332:refnum<k21>, "error out"=w329:errorcluster)  [unwired: 9 in, 1 out]
          n170 = Unbundle By Name(w329) -> ("status"=w328:bool)
          n171 = Or(x=w328, y=w326) -> (x .or. y?=w327:bool)
        }
        n172 = call <vilib>:"DAQmx Stop Task.vi"("task/channels in"=w317, "error in"=w320) -> ("task out"=w318:refnum<k21>, "error out"=w319:errorcluster)  [unwired: 12 in]
        n173 = call <vilib>:"DAQmx Clear Task.vi"("task in"=w318, "error in"=w319) -> ("error out"=w314:errorcluster)  [unwired: 13 in]
        n174 = call <vilib>:"Simple Error Handler.vi"("type of dialog (OK msg:1)"=w313, "error in (no error)"=w314) -> ()  [unwired: 3 in, 5 out]
      }
      event "启用抓取控制1-3-4": Value Change {
        w344 = T1 3 items=["无对话框", "确定信息", "继续或停止信息", "确定信息＋警告", "继续/停止＋警告"] ("对话框类型（确定信息：1）")
        # "停止清除"
        # "通道设置"
        # "机械手抓放控制"
        n175 = event-data() -> ()  [unwired: 1 in, 6 out]
        n176 = call-poly <vilib>:"DAQmx Create Virtual Channel.vi"("maximum value"="maximum value 7", "minimum value"=0.0 ("minimum value 2"), "physical channels"=tag "Dev1/ao0, Dev1/ao2:3") -> ("task out"=w346:refnum<k21>, "error out"=w353:errorcluster)  [unwired: 11 in]
        n177 = call <vilib>:"DAQmx Start Task.vi"("task/channels in"=w346, "error in"=w353) -> ("task out"=w347:refnum<k21>, "error out"=w352:errorcluster)  [unwired: 12 in]
        n178 = while {
          tunnel: w347 -> [w364]
          tunnel: [w363] -> w348
          tunnel: w352 -> [w362]
          tunnel: [w360] -> w351
          stop <- w358 stop-if-true
          # "输出"
          # "输出电压值设置"
          n179 = event shown="[4] \"总停止按钮\": 值改变" {
            selector: _ -> [_ _ _ _ _]
            dyn-events: _ -> [_ _ _ _ _]
            timeout: _ -> [_ _ _ _ _]
            tunnel: [_ 10.0 ("data") 1.0 ("data") 1.0 ("data") 1.0 ("data")] -> w356
            tunnel: [_ FALSE FALSE "无极控制停止按钮 1-3-4" TRUE] -> w357
            event Timeout {
              n180 = event-data() -> ()  [unwired: 1 in, 3 out]
            }
            event "抓取1-4": Value Change {
              n181 = event-data() -> ()  [unwired: 1 in, 4 out]
            }
            event "释放 1-3-4": Value Change {
              n182 = event-data() -> ()  [unwired: 1 in, 4 out]
            }
            event "无极控制停止按钮 1-3-4": Value Change {
              n183 = event-data() -> ()  [unwired: 1 in, 4 out]
            }
            event "总停止按钮": Value Change {
              n184 = event-data() -> ()  [unwired: 1 in, 4 out]
            }
          }
          n185 = Build Array(w356, w356, w356) -> (w355:dbl[])
          n186 = call-poly <vilib>:"DAQmx Write.vi"("task/channels in"=w364, "auto start"=FALSE, "data"=w355, "error in"=w362) -> ("task out"=w363:refnum<k21>, "error out"=w360:errorcluster)  [unwired: 9 in, 1 out]
          n187 = Unbundle By Name(w360) -> ("status"=w359:bool)
          n188 = Or(x=w359, y=w357) -> (x .or. y?=w358:bool)
        }
        n189 = call <vilib>:"DAQmx Stop Task.vi"("task/channels in"=w348, "error in"=w351) -> ("task out"=w349:refnum<k21>, "error out"=w350:errorcluster)  [unwired: 12 in]
        n190 = call <vilib>:"DAQmx Clear Task.vi"("task in"=w349, "error in"=w350) -> ("error out"=w345:errorcluster)  [unwired: 13 in]
        n191 = call <vilib>:"Simple Error Handler.vi"("type of dialog (OK msg:1)"=w344, "error in (no error)"=w345) -> ()  [unwired: 3 in, 5 out]
      }
      event "总停止按钮": Value Change {
        n192 = event-data() -> ()  [unwired: 1 in, 6 out]
      }
    }
    n193 = Wait (ms)(milliseconds to wait=u32 100 ("等待时间（毫秒）")) -> ()  [unwired: 1 out]
  }
